vi "detect_0102.vi"(8 "error in (no error)":errorcluster, 11 "VISA Refnum in":refnum<visa-resource-name>) -> (0 "error out":errorcluster, 1 "RECEIVED":bool, 2 "NOT RECEIVED":bool, 3 "VISA Refnum out":refnum<visa-resource-name>)   [LabVIEW 2019]
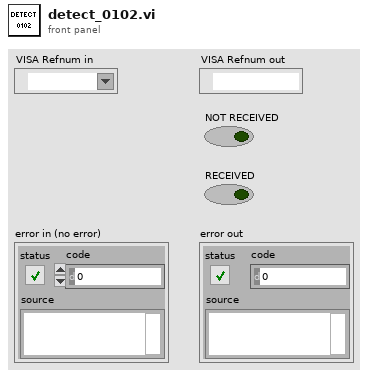
[diagram p1: front panel]
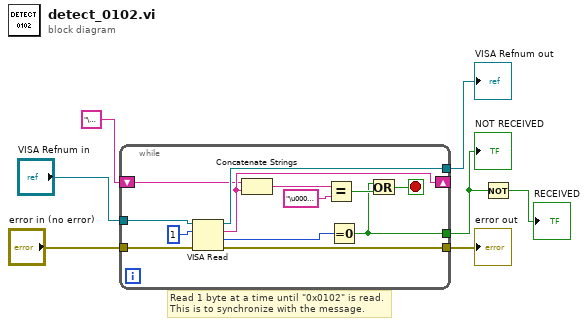
[diagram p0: block diagram]
diagram:
  # "Read 1 byte at a time until \"0x0102\" is read.\nThis is to synchronize with the message."
  n1 = while {
    tunnel: "VISA Refnum in" -> [w18]
    tunnel: "error in (no error)" -> [w20]
    tunnel: [w19] -> w2
    tunnel: [w15] -> w1
    shift-right: [w13] -> _
    shift-left: "\u0000" ("read buffer") -> [w12]
    tunnel: [w8] -> w6
    stop <- w10 stop-if-true
    n2 = VISA Read(VISA resource name=w18, byte count=u32 1, error in (no error)=w20) -> (VISA resource name out=w15:refnum<visa-resource-name>, read buffer=w13:string, return count=w9:u32, error out=w19:errorcluster)
    n3 = Concatenate Strings(w12, w13) -> (w14:string)
    n4 = Equal?(x=w14, y="\u0001\u0002") -> (x = y?=w11:bool)
    n5 = Equal To 0?(x=w9) -> (x = 0?=w8:bool)
    n6 = Or(x=w8, y=w11) -> (x .or. y?=w10:bool)
  }
  "NOT RECEIVED" <- w6
  "error out" <- w2
  "VISA Refnum out" <- w1
  n7 = Not(x=w6) -> (.not. x?=→"RECEIVED":bool)
